vi "Insert User Operation his.vi"(8 "data":string, 9 "event":string, 10 "account":string, 11 "DBlink":string="Driver={ODBC Driver 17 for SQL Server};Server=localhost\\SQLEXPRESS;Database=ZDX201;UID=labview;PWD=Dsa@54137926") -> (0 "error out":errorcluster)   [LabVIEW 2019]
uses:
  <vilib>/addons/database/Connection.llb/DB Tools Open Connec (String).vi
  <vilib>/addons/database/NI_Database_API.lvlib
panel:
  in  "Insert value":T1={"account"="DSA", "create_time"=timestamp(3727229595.4569273 s since 1904-01-01), "event"="運作紀錄 - 總次數歸零", "data"="運作紀錄 - 總次數歸零"}
  in  "columns":string[](array[string])=["account", "create_time", "event", "data"]
  in  "error in (no error)":errorcluster
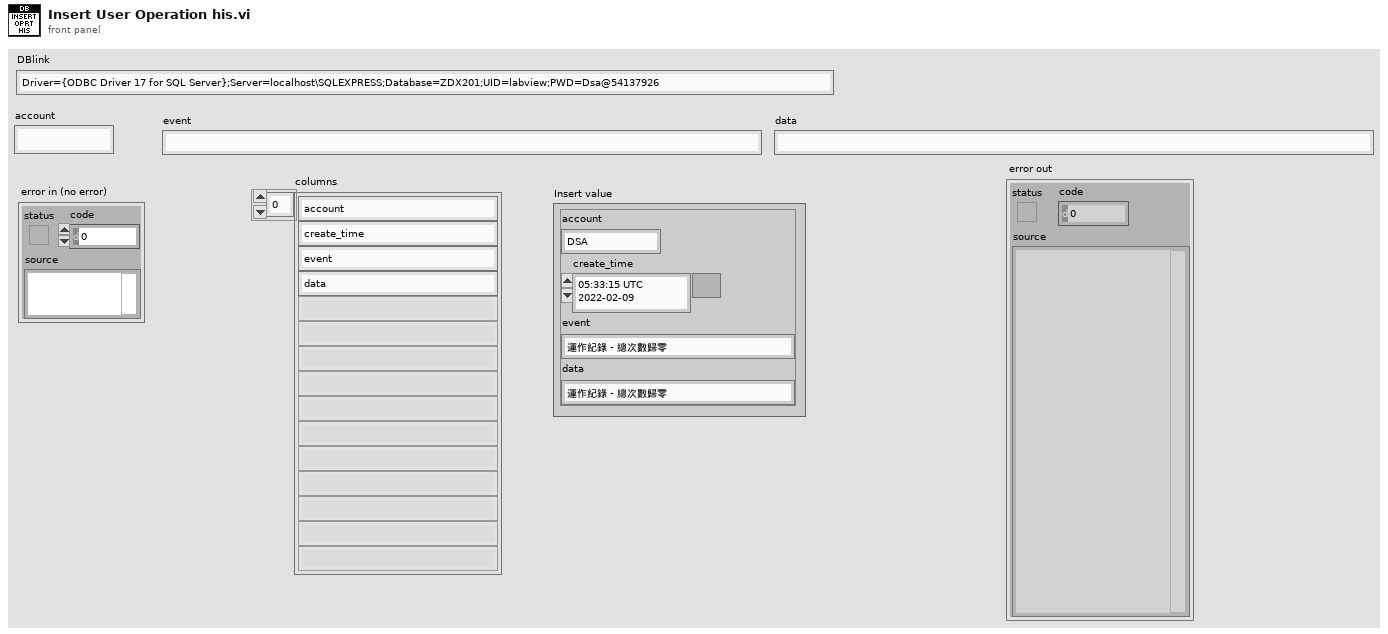
[diagram p1: front panel]
types:
  T1 = cluster{"account":string, "create_time":timestamp, "event":string, "data":string}
  T2 = typedef "NI_Database_API.lvlib/Conn ObjectReference.ctl" = refnum<k1>
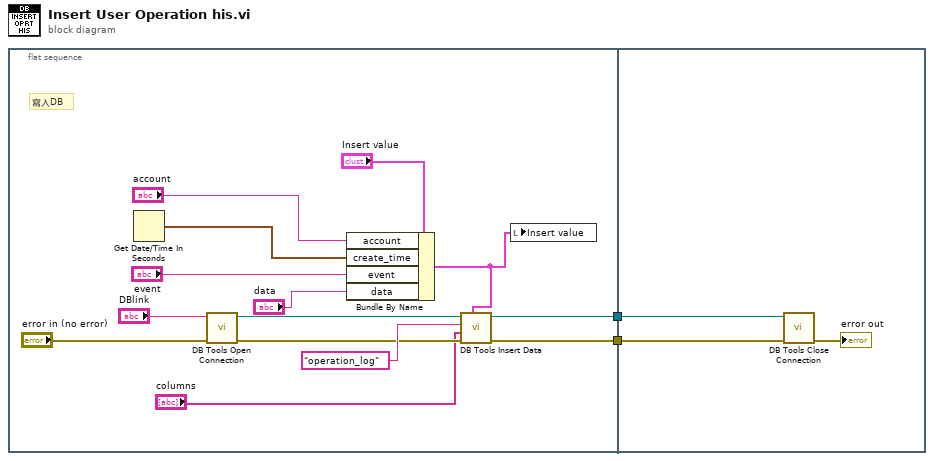
[diagram p0: block diagram]
diagram:
  n1 = flat-sequence {
    tunnel: [w14] -> w2
    tunnel: [w15] -> w1
    tunnel: w2 -> [w17]
    tunnel: w1 -> [w18]
    frame #0 {
      # "寫入DB"
      n2 = Get Date/Time In Seconds() -> (seconds since 1Jan1904=w5:timestamp)
      n3 = call-poly <vilib>:"DB Tools Open Connection.vi"("error in (no error)"="error in (no error)", "connection information"="DBlink") -> ("error out"=w12:errorcluster, "connection reference"=w11:T2)  [unwired: 6 in]
      n4 = Bundle By Name(cluster="Insert value", "account"="account", "create_time"=w5, "event"="event", "data"="data") -> (w4:T1)
      n5 = call <vilib>:"DB Tools Insert Data.vi"("data"=w4, "error in (no error)"=w12, "columns"="columns", "table"="operation_log", "connection reference"=w11) -> ("error out"=w14:errorcluster, "connection reference out"=w15:T2)  [unwired: 5 in]
      n6 = local write "Insert value"(w4) -> ()
    }
    frame #1 {
      n7 = call <vilib>:"DB Tools Close Connection.vi"("error in (no error)"=w17, "connection reference"=w18) -> ("error out"=→"error out":errorcluster)  [unwired: 5 in]
    }
  }
